vi "main_check.vi"() -> ()   [LabVIEW 2020]
uses:
  <vilib>/DAQmx/create/channels.llb/DAQmx Create Channel (DO-Digital Output).vi
  <vilib>/DAQmx/create/channels.llb/DAQmx Create Channel (DI-Digital Input).vi
panel:
  out "Boolean array":bool[](array[boolean])
  in  "Read Pin":tag="Dev1/port0/line0:7"
  in  "Clear Pin":tag="Dev1/port0/line0:7"
  in  "Sync Pin":tag="Dev1/port0/line0:7"
  in  "Data Pin":tag="Dev1/port0/line0:7"
  in  "Write Pin":tag="Dev1/port0/line0:7"
  # "___"
  # "___"
  # "___"
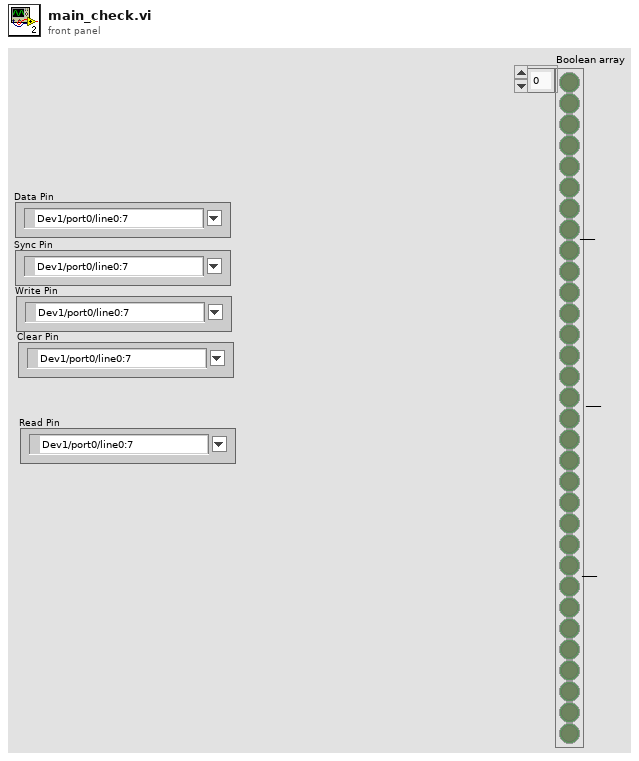
[diagram p1: front panel]
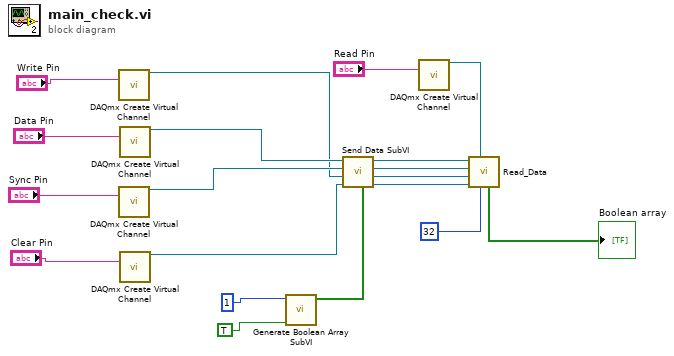
[diagram p0: block diagram]
diagram:
  n1 = call-poly <vilib>:"DAQmx Create Virtual Channel.vi"("lines"="Write Pin") -> ("task out"=w2:refnum<k21>)  [unwired: 13 in, 1 out]
  n2 = call-poly <vilib>:"DAQmx Create Virtual Channel.vi"("lines"="Sync Pin") -> ("task out"=w3:refnum<k21>)  [unwired: 13 in, 1 out]
  n3 = call-poly <vilib>:"DAQmx Create Virtual Channel.vi"("lines"="Data Pin") -> ("task out"=w4:refnum<k21>)  [unwired: 13 in, 1 out]
  n4 = call-poly <vilib>:"DAQmx Create Virtual Channel.vi"("lines"="Clear Pin") -> ("task out"=w1:refnum<k21>)  [unwired: 13 in, 1 out]
  n5 = call "Generate Boolean Array SubVI.vi"("Activate: 1\nDeactivate: 0"=TRUE, "Tube"=1) -> ("Boolean array"=w17:bool[])  [unwired: 9 in]
  n6 = call "Send Data SubVI.vi"("Data Pin Task In"=w4, "Sync Pin Task In"=w3, "Write Pin Task In"=w2, "Clear Pin Task In"=w1, "Data"=w17) -> ("Data Pin Task Out"=w11:refnum<k21>, "Sync Pin Task Out"=w10:refnum<k21>, "Write Pin Task Out"=w9:refnum<k21>, "Clear Pin Task Out"=w8:refnum<k21>)  [unwired: 1 in]
  n7 = call-poly <vilib>:"DAQmx Create Virtual Channel.vi"("lines"="Read Pin") -> ("task out"=w7:refnum<k21>)  [unwired: 13 in, 1 out]
  n8 = call "Read_Data.vi"("Bits in Register"=32, "Read Pin Task In"=w7, "Clear Pin Task In"=w8, "Sync Pin Task In"=w9, "Data Pin Task In"=w10, "Write Pin Task In"=w11) -> ("Boolean array"=→"Boolean array":bool[])  [unwired: 5 out]
